vi "Test Sampling.vi"(8 "error in (no error)":errorcluster, 11 "Instrument.Lockin in":refnum<class "Instrument.Lockin.lvclass">) -> (0 "error out":errorcluster, 3 "Instrument.Lockin out":refnum<class "Instrument.Lockin.lvclass">)   [LabVIEW 2019]
uses:
  src/Instrument.Lockin/Instrument.Lockin.lvclass
  src/Instrument.DAQ/Typedefs/DAQ.Sampling.Sampling--Cluster.ctl
  src/Instrument.DAQ/Typedefs/DAQ.Sampling.Fs Mode--enum.ctl
  <userlib>/_OpenG.lib/numeric/numeric.llb/Random Number Within Range - DBL__ogtk.vi
  <userlib>/_OpenG.lib/numeric/numeric.llb/Random Number Within Range - I32__ogtk.vi
  <vilib>/addons/_JKI Toolkits/Caraya/classes/Assert/Assert Almost Equal_Float.vi
  <vilib>/addons/_JKI Toolkits/Caraya/classes/Test/Test.lvclass
  <vilib>/addons/_JKI Toolkits/Caraya/classes/Assert/Assert.lvclass
  src/Instrument.DAQ/Instrument.DAQ.lvclass
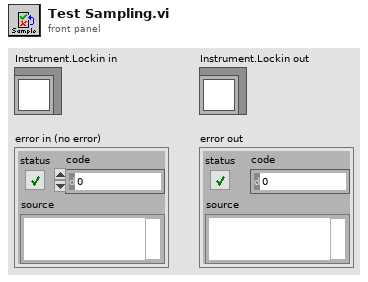
[diagram p1: front panel]
types:
  T1 = typedef "Instrument.Lockin.lvlib/Instrument.DAQ.lvclass/DAQ.Sampling.Sampling--Cluster.ctl" = cluster{"Fs":dbl, "#s":i32}
  T2 = typedef "Instrument.Lockin.lvlib/Instrument.DAQ.lvclass/DAQ.Sampling.Fs Mode--enum.ctl" = enum16{"Manual", "Auto Fs", "Max Fs"}
  T3 = typedef "Instrument.LockinAPI.lvclass/LockinAPI.Sampling.Sampling--Cluster.ctl" = cluster{"Fs":dbl, "#s":i32}
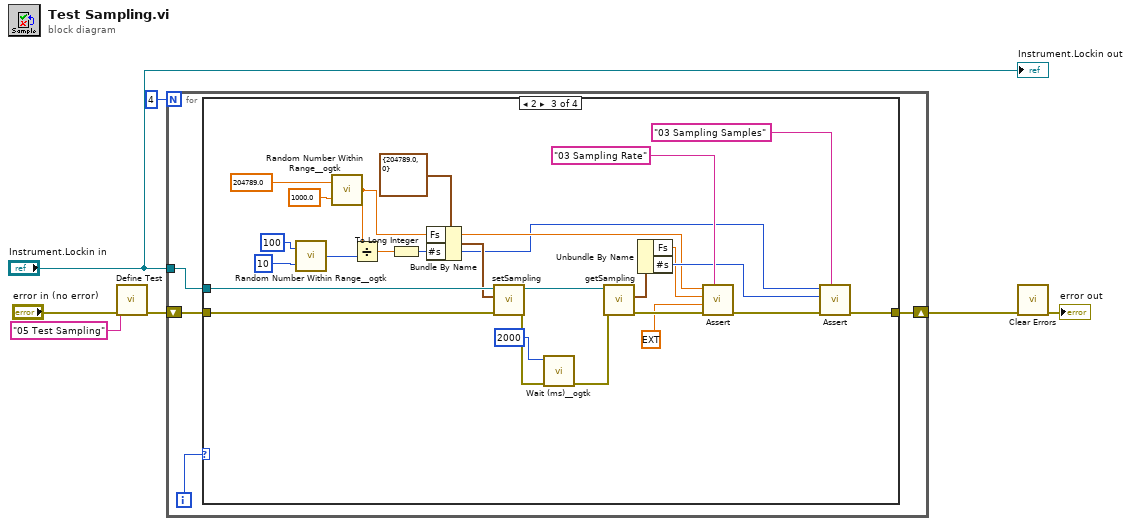
[diagram p0: block diagram]
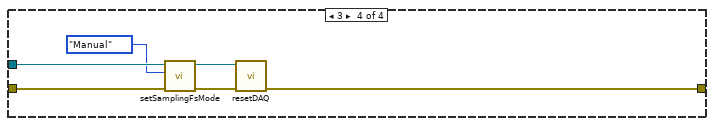
[diagram p4: hidden frame]
diagram:
  n1 = call <vilib>:"Define Test.vi"("error in (no error)"="error in (no error)", "Label (VI Title)"="05 Test Sampling") -> ("error out"=w5:errorcluster)  [unwired: 8 in, 1 out]
  n2 = for {
    N: 4 -> [_]
    tunnel: "Instrument.Lockin in" -> [w9]
    shift-right: [w8] -> w2
    shift-left: w5 -> [w10]
    i -> [w11]
    n3 = case shown="2" w11 {
      tunnel: w10 -> [w12 w13 w29 w42]
      tunnel: w9 -> [_ _ w30 w41]
      tunnel: [w12 w13 w24 w40] -> w8
      frame 0, Default {
      }
      frame 1 {
      }
      frame 2 {
        n4 = call-poly <userlib>:"Random Number Within Range__ogtk.vi"("High"=u32 100, "Low"=u32 10) -> ("Random Number"=w28:i32)  [unwired: 3 in]
        n5 = call-poly <userlib>:"Random Number Within Range__ogtk.vi"("High"=204789.0, "Low"=1000.0) -> ("Random Number"=w20:dbl)  [unwired: 3 in]
        n6 = Divide(x=w20, y=w28) -> (x/y=w21:dbl)
        n7 = To Long Integer(number=w21) -> (32bit integer=w16:i32)
        n8 = Bundle By Name(cluster=T1 {"Fs"=204789.0, "#s"=0} ("sampling"), "Fs"=w20, "#s"=w16) -> (w27:T1)
        n9 = call-dynamic "setSampling.vi"("error in (no error)"=w29, "sampling"=w27, "Instrument.Lockin in"=w30) -> ("error out"=w18:errorcluster, "Instrument.Lockin out"=w33:refnum<class "Instrument.Lockin.lvclass">)  [unwired: 7 in]
        n10 = call <userlib>:"Wait (ms)__ogtk.vi"("error in (no error)"=w18, "milliseconds to wait"=u32 2000) -> ("error out"=w15:errorcluster)  [unwired: 8 in, 1 out]
        n11 = call-dynamic "getSampling.vi"("error in (no error)"=w15, "Instrument.Lockin in"=w33) -> ("error out"=w31:errorcluster, "sampling"=w23:T3)  [unwired: 7 in, 1 out]
        n12 = Unbundle By Name(w23) -> ("Fs"=w19:dbl, "#s"=w22:i32)
        n13 = call-poly <vilib>:"Assert.vi"("Label"="03 Sampling Rate", "error in (no error)"=w31, "Tolerance"=ext 1.0, "Actual"=w19, "Expected"=w20) -> ("error out"=w25:errorcluster)  [unwired: 5 in, 1 out]
        n14 = call-poly <vilib>:"Assert.vi"("Label"="03 Sampling Samples", "error in (no error)"=w25, "Actual"=w22, "Expected"=w16) -> ("error out"=w24:errorcluster)  [unwired: 6 in, 1 out]
      }
      frame 3 {
        n15 = call-dynamic "setSamplingFsMode.vi"("error in (no error)"=w42, "Fs Mode"=DAQ.Sampling.Fs_Mode--enum."Manual" ("Sampling Mode"), "Instrument.Lockin in"=w41) -> ("error out"=w43:errorcluster, "Instrument.Lockin out"=w44:refnum<class "Instrument.Lockin.lvclass">)  [unwired: 7 in]
        n16 = call-dynamic "resetDAQ.vi"("error in (no error)"=w43, "Instrument.Lockin in"=w44) -> ("error out"=w40:errorcluster)  [unwired: 8 in, 1 out]
      }
    }
  }
  n17 = call <vilib>:"Clear Errors.vi"("error in (no error)"=w2) -> ("error out"=→"error out":errorcluster)  [unwired: 5 in, 1 out]
  "Instrument.Lockin out" <- "Instrument.Lockin in"
